vi "Anritsu VNA Read Identification.vi"(8 "error in (no error)":errorcluster, 11 "VISA Resource Name":refnum<visa-resource-name>) -> (0 "error out":errorcluster, 1 "Serial Number":string, 2 "Model Number":string, 3 "dup VISA Resource Name":refnum<visa-resource-name>, 5 "Firmware":string)   [LabVIEW 2011]
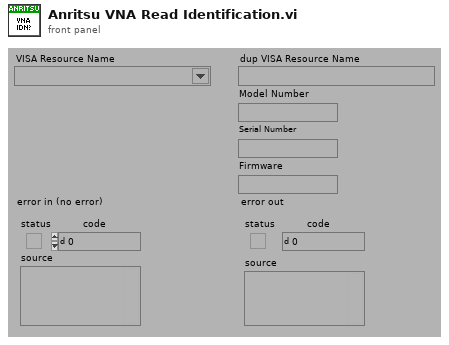
[diagram p1: front panel]
types:
  T1 = typedef "Anritsu VNA Model.ctl" = enum16{"Not Supported", "37XXXX", "MS20XXX", "MS462XX", "MS464XX"}
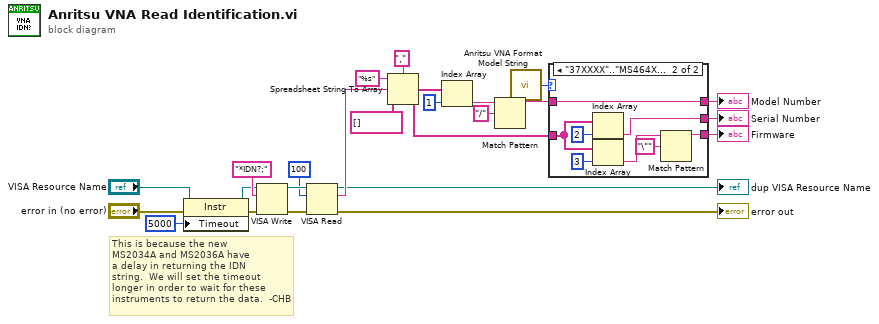
[diagram p0: block diagram]
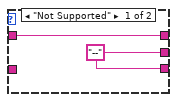
[diagram p2: hidden frame]
diagram:
  # "This is because the new\nMS2034A and MS2036A have\na delay in returning the IDN\nstring.  We will set the timeout\nlonger in order to wait for these\ninstruments to return the data.  -CHB"
  n1 = property class="Instr"(reference="VISA Resource Name", error in="error in (no error)", "Timeout"=u32 5000 ("General Settings:Timeout Value")) -> (reference out=w8:refnum<visa-resource-name>, error out=w3:errorcluster)
  n2 = VISA Write(VISA resource name=w8, write buffer="*IDN?;", error in (no error)=w3) -> (VISA resource name out=w24:refnum<visa-resource-name>, error out=w11:errorcluster)  [unwired: 1 out]
  n3 = VISA Read(VISA resource name=w24, byte count=u32 100, error in (no error)=w11) -> (VISA resource name out=→"dup VISA Resource Name":refnum<visa-resource-name>, read buffer=w7:string, error out=→"error out":errorcluster)  [unwired: 1 out]
  n4 = Spreadsheet String To Array(delimiter (Tab)=",", format string="%s", spreadsheet string=w7, array type (2D Dbl)=string[] []) -> (array=w17:string[])
  n5 = Index Array(array=w17, index=1) -> (element=w12:string)
  n6 = Match Pattern(string=w12, regular expression="/") -> (before substring=w1:string)  [unwired: 4 out]
  n7 = call "Anritsu VNA Format Model String.vi"("Model"=w1) -> ("Model"=w2:T1)
  n8 = case shown="\"37XXXX\"..\"MS464XX\"" w2 {
    tunnel: [w25 w27] -> w16
    tunnel: w17 -> [_ w32]
    tunnel: [w26 w31] -> w15
    tunnel: [w26 w28] -> w14
    tunnel: w1 -> [w25 w27]
    frame "Not Supported" {
      w26 = "--"
    }
    frame "37XXXX".."MS464XX" {
      n9 = Index Array(array=w32, index=2) -> (element=w31:string)
      n10 = Index Array(array=w32, index=3) -> (element=w29:string)
      n11 = Match Pattern(string=w29, regular expression="\"") -> (before substring=w28:string)  [unwired: 4 out]
    }
  }
  "Model Number" <- w16
  "Serial Number" <- w15
  "Firmware" <- w14
